vi "TCP - Transfer Groups to DSF Cluster.vi"(0 "local address":string, 1 "local port":string, 2 "Transfer Groups":T1[](array[typedef]) {"transfers"."channels"."core"."string offset" format="%d bytes"}) -> (16 "DSF Cluster":T12)   [LabVIEW 2024]
uses:
  <vilib>/addons/VeriStand Custom Device Scripting APIs/Data Sharing Framework/DSF Core.lvlibp/Typedefs/DSF Engine Framework Configuration.ctl
  <vilib>/addons/VeriStand Custom Device Scripting APIs/Data Sharing Framework/DSF Core.lvlibp/Typedefs/DSF Engine Plugin Configuration.ctl
  <vilib>/addons/VeriStand Custom Device Scripting APIs/Data Sharing Framework/DSF Core.lvlibp/Typedefs/Core Plugin Configuration.ctl
  <vilib>/addons/VeriStand Custom Device Scripting APIs/Data Sharing Framework/DSF Core.lvlibp/Typedefs/DSF Timing Info.ctl
  <vilib>/addons/VeriStand Custom Device Scripting APIs/Data Sharing Framework/DSF Core.lvlibp/Typedefs/DSF Settings Info.ctl
  <vilib>/addons/VeriStand Custom Device Scripting APIs/Data Sharing Framework/DSF Core.lvlibp/Typedefs/DSF Engine Plugin Thread Configuration.ctl
  <vilib>/addons/VeriStand Custom Device Scripting APIs/Data Sharing Framework/DSF Core.lvlibp/Typedefs/Core Thread Configuration.ctl
  <vilib>/addons/VeriStand Custom Device Scripting APIs/Data Sharing Framework/DSF Core.lvlibp/Typedefs/DSF Engine Transfer Group Configuration.ctl
  <vilib>/addons/VeriStand Custom Device Scripting APIs/Data Sharing Framework/DSF Core.lvlibp/Typedefs/Core Group Configuration.ctl
  <vilib>/addons/VeriStand Custom Device Scripting APIs/Data Sharing Framework/DSF Core.lvlibp/Typedefs/DSF Direction.ctl
  <vilib>/addons/VeriStand Custom Device Scripting APIs/Data Sharing Framework/DSF Core.lvlibp/Typedefs/DSF Timeout Behavior.ctl
  <vilib>/addons/VeriStand Custom Device Scripting APIs/Data Sharing Framework/DSF Core.lvlibp/Typedefs/DSF Engine Transfer Configuration.ctl
  <vilib>/addons/VeriStand Custom Device Scripting APIs/Data Sharing Framework/DSF Core.lvlibp/Typedefs/Core Transfer Configuration.ctl
  <vilib>/addons/VeriStand Custom Device Scripting APIs/Data Sharing Framework/DSF Core.lvlibp/Typedefs/DSF Engine Channel Configuration.ctl
  <vilib>/addons/VeriStand Custom Device Scripting APIs/Data Sharing Framework/DSF Core.lvlibp/Typedefs/Core Channel Configuration.ctl
  <vilib>/addons/VeriStand Custom Device Scripting APIs/Data Sharing Framework/DSF Core.lvlibp/Typedefs/DSF Data Type.ctl
  <vilib>/addons/VeriStand Custom Device Scripting APIs/Data Sharing Framework/DSF Core.lvlibp
  <vilib>/addons/VeriStand Custom Device Scripting APIs/Data Sharing Framework/DSF Core.lvlibp/Classes/Configuration/Core/Channel/Channel Configuration.lvclass
  <vilib>/addons/VeriStand Custom Device Scripting APIs/Data Sharing Framework/DSF Core.lvlibp/Classes/Configuration/Core/Transfer/Transfer Configuration.lvclass
  <vilib>/addons/VeriStand Custom Device Scripting APIs/Data Sharing Framework/DSF Core.lvlibp/Classes/Configuration/Core/Group/Group Configuration.lvclass
  <vilib>/addons/VeriStand Custom Device Scripting APIs/Data Sharing Framework/DSF Core.lvlibp/Classes/Configuration/Core/Thread/Thread Configuration.lvclass
  <vilib>/addons/VeriStand Custom Device Scripting APIs/Data Sharing Framework/DSF Core.lvlibp/Classes/Configuration/Core/Plugin/Plugin Configuration.lvclass
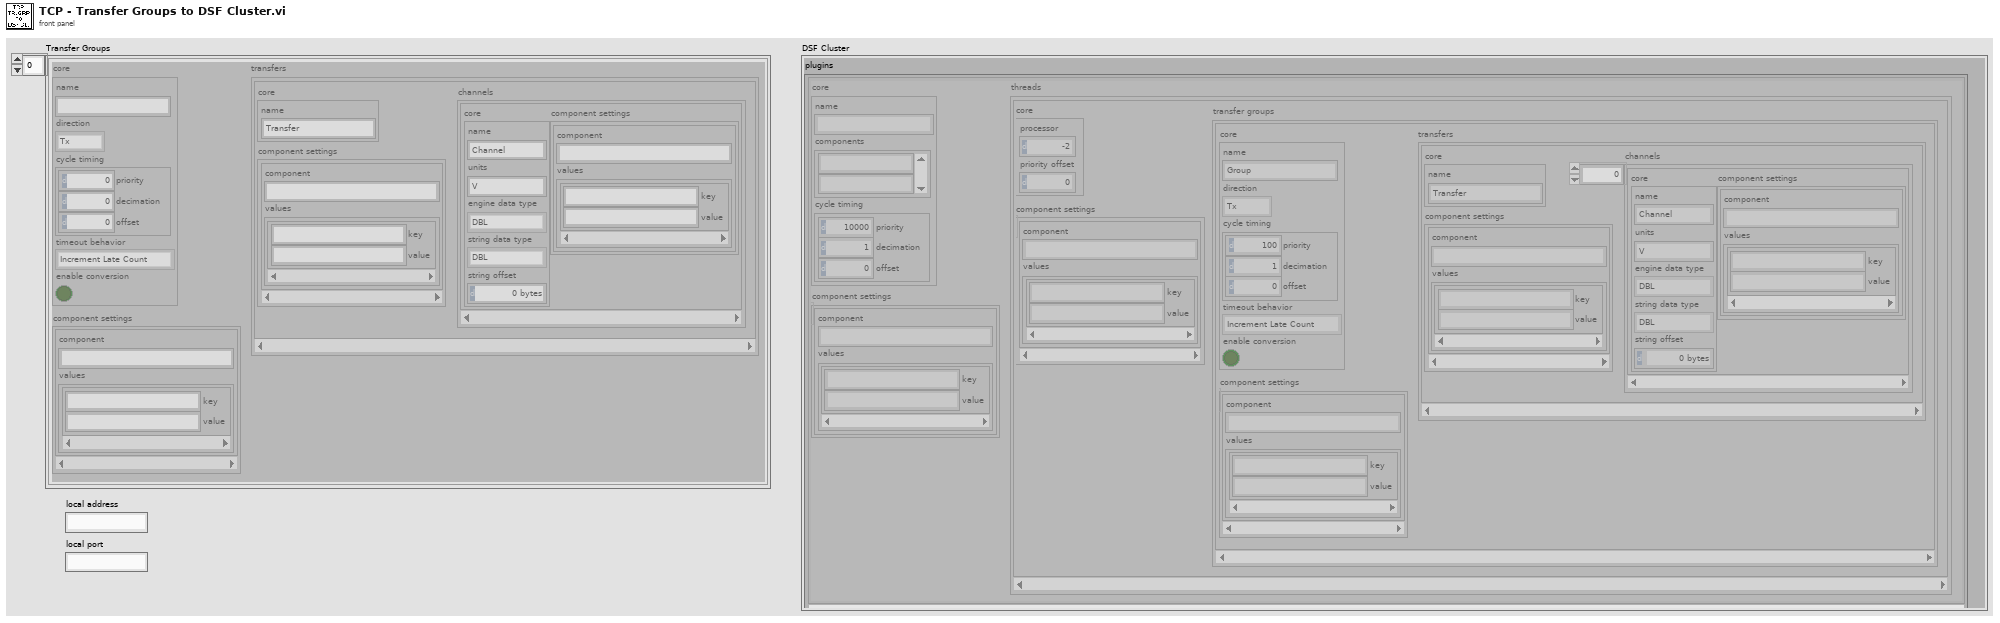
[diagram p1: front panel]
types:
  T1 = typedef "DSF Core.lvlibp/DSF Engine Transfer Group Configuration.ctl" = cluster{"core":T2, "component settings":T6[], "transfers":T7[]}
  T2 = typedef "DSF Core.lvlibp/Group Configuration.lvclass/Core Group Configuration.ctl" = cluster{"name":string, "direction":T3, "cycle timing":T4, "timeout behavior":T5, "enable conversion":bool}
  T3 = typedef "DSF Core.lvlibp/DSF Direction.ctl" = enum8{"Tx", "Rx"}
  T4 = typedef "DSF Core.lvlibp/DSF Timing Info.ctl" = cluster{"priority":u64, "decimation":u64, "offset":u64}
  T5 = typedef "DSF Core.lvlibp/DSF Timeout Behavior.ctl" = enum8{"Increment Late Count", "Throw Error"}
  T6 = typedef "DSF Core.lvlibp/DSF Settings Info.ctl" = cluster{"component":string, "values":cluster{"key":string, "value":string}[]}
  T7 = typedef "DSF Core.lvlibp/DSF Engine Transfer Configuration.ctl" = cluster{"core":T8, "component settings":T6[], "channels":T9[]}
  T8 = typedef "DSF Core.lvlibp/Transfer Configuration.lvclass/Core Transfer Configuration.ctl" = cluster{"name":string}
  T9 = typedef "DSF Core.lvlibp/DSF Engine Channel Configuration.ctl" = cluster{"core":T10, "component settings":T6[]}
  T10 = typedef "DSF Core.lvlibp/Channel Configuration.lvclass/Core Channel Configuration.ctl" = cluster{"name":string, "units":string, "engine data type":T11, "string data type":T11, "string offset":u64}
  T11 = typedef "DSF Core.lvlibp/DSF Data Type.ctl" = enum8{"Bool", "SGL", "DBL", "I8", "I16", "I32", "I64", "U8", "U16", "U32", "U64"}
  T12 = typedef "DSF Core.lvlibp/DSF Engine Framework Configuration.ctl" = cluster{"plugins":T13[]}
  T13 = typedef "DSF Core.lvlibp/DSF Engine Plugin Configuration.ctl" = cluster{"core":T14, "component settings":T6[], "threads":T15[]}
  T14 = typedef "DSF Core.lvlibp/Plugin Configuration.lvclass/Core Plugin Configuration.ctl" = cluster{"name":string, "components":string[], "cycle timing":T4}
  T15 = typedef "DSF Core.lvlibp/DSF Engine Plugin Thread Configuration.ctl" = cluster{"core":T16, "component settings":T6[], "transfer groups":T1[]}
  T16 = typedef "DSF Core.lvlibp/Thread Configuration.lvclass/Core Thread Configuration.ctl" = cluster{"processor":i32, "priority offset":i16}
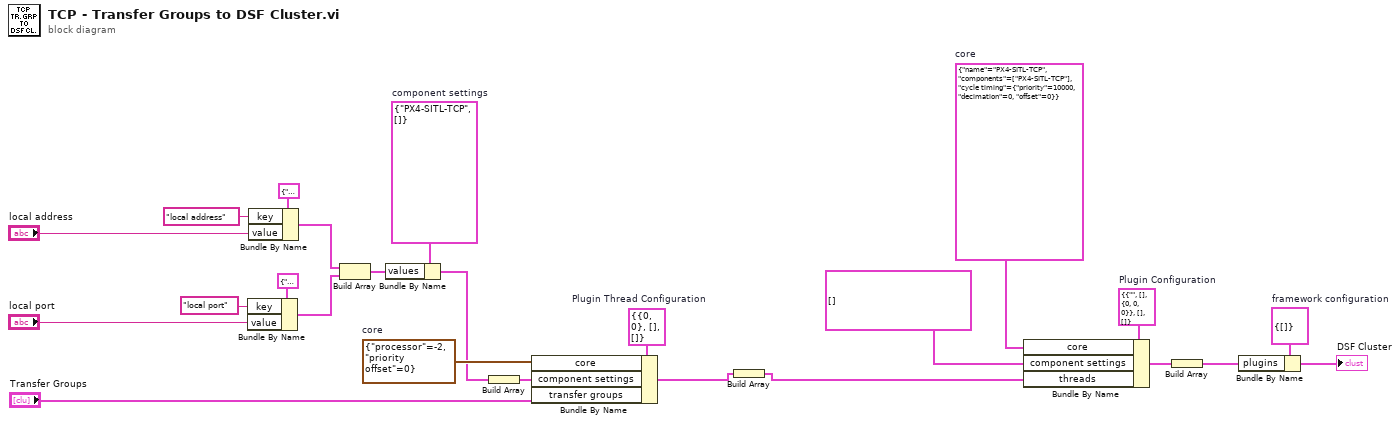
[diagram p0: block diagram]
diagram:
  w7 = T16 {"processor"=-2, "priority offset"=0}  # core
  w6 = T15 {"core"={"processor"=0, "priority offset"=0}, "component settings"=[], "transfer groups"=[]}  # Plugin Thread Configuration
  w9 = T6 {"component"="PX4-SITL-TCP", "values"=[]}  # component settings
  w19 = T14 {"name"="PX4-SITL-TCP", "components"=["PX4-SITL-TCP"], "cycle timing"={"priority"=10000, "decimation"=0, "offset"=0}}  # core
  w22 = T13 {"core"={"name"="", "components"=[], "cycle timing"={"priority"=0, "decimation"=0, "offset"=0}}, "component settings"=[], "threads"=[]}  # Plugin Configuration
  w24 = T12 {"plugins"=[]}  # framework configuration
  n1 = Bundle By Name(cluster=cluster{"key":string, "value":string} {"key"="", "value"=""} ("setting"), "key"="local port", "value"="local port") -> (w10:cluster{"key":string, "value":string})
  n2 = Bundle By Name(cluster=cluster{"key":string, "value":string} {"key"="", "value"=""} ("setting"), "key"="local address", "value"="local address") -> (w11:cluster{"key":string, "value":string})
  n3 = Build Array(w11, w10) -> (w8:cluster{"key":string, "value":string}[])
  n4 = Bundle By Name(cluster=w9, "values"=w8) -> (w5:T6)
  n5 = Build Array(w5) -> (w4:T6[])
  n6 = Bundle By Name(cluster=w6, "core"=w7, "component settings"=w4, "transfer groups"="Transfer Groups") -> (w2:T15)
  n7 = Build Array(w2) -> (w1:T15[])
  n8 = Bundle By Name(cluster=w22, "core"=w19, "component settings"=T6[] [], "threads"=w1) -> (w21:T13)
  n9 = Build Array(w21) -> (w23:T13[])
  n10 = Bundle By Name(cluster=w24, "plugins"=w23) -> (→"DSF Cluster":T12)
